vi "AudioTest.Config, Read_Write Microphone Test Setup.vi"(7 "Read(F)/Write(T)":bool, 8 "error in (no error)":errorcluster, 10 "Params":T6={"Devices"={"AudioOutName"="Line", "AudioInName"="HMD"}, "SweepParams"={"Duration"=2.0, "Amplitude"=1.0, "FreqStart"=20.0, "FreqEnd"=20000.0, "SampleRate"=44100.0, "StepCnt"=120, "FreqSpacing"=enum."Logarithmic", "Settling"={"Time"=0.0, "Cycles"=1.0}, "Measurement"={"Time"=0.001, "Cycles"=10.0}, "SyncPulseEn"=FALSE}, "DataFolder"=path "C:/MTE/Utah Core Audio Test/Data", "AvgLevelParams"={"Freq Start"=20.0, "Freq End"=20000.0}, "Limits"={"CoveredMicAttn_dB"=500.0, "AvgLevelLL_dBFS"=12000.0, "AvgLevelUL_dBFS"=44100.0, "FreqRespLim"=path "C:/MTE/Utah Core Audio Test/Config/Microphone Test Freq Response Limits.ini", "THDLim"=path "C:/MTE/Utah Core Audio Test/Config/Microphone Test THD Limits.ini"}, "SpeakerCalFile"=path "C:/MTE/Utah Core Audio Test/Config/Microphone Test Speaker Calibration.ini", "Volume"=0.0} {"SweepParams"."Measurement"."Cycles" min=5.0 max=1000.0 step=1.0; "SweepParams"."Measurement"."Time" min=0.0 max=5.0 step=0.0001 format="%.3f s"; "SweepParams"."Settling"."Cycles" min=0.0 max=100.0 step=0.5; "SweepParams"."Settling"."Time" min=0.0 max=5.0 step=0.0001 format="%.3f s"; "SweepParams"."StepCnt" min=1; "SweepParams"."Amplitude" min=0.0 max=1.0 step=0.1}, 11 "Config Folder":path=path "C:/MTE/Utah Core Audio Test/Config") -> (0 "error out":errorcluster, 2 "Params":T5={"Devices"={"AudioOutName"="Line", "AudioInName"="HMD"}, "SweepParams"={"Duration"=2.0, "Amplitude"=1.0, "FreqStart"=20.0, "FreqEnd"=20000.0, "SampleRate"=44100.0, "StepCnt"=120, "FreqSpacing"=enum."Logarithmic", "Settling"={"Time"=0.0, "Cycles"=1.0}, "Measurement"={"Time"=0.001, "Cycles"=10.0}, "SyncPulseEn"=FALSE}, "DataFolder"=path "C:/MTE/Utah Core Audio Test/Data", "AvgLevelParams"={"Freq Start"=20.0, "Freq End"=20000.0}, "BlockedMicLim"={"CoveredMicAttn_dB"=500.0, "AvgLevelLL_dBFS"=12000.0, "AvgLevelUL_dBFS"=44100.0, "FreqRespLim"=path "C:/MTE/Utah Core Audio Test/Config/Microphone Test Freq Response Limits.ini", "THDLim"=path "C:/MTE/Utah Core Audio Test/Config/Microphone Test THD Limits.ini"}, "SpeakerCalFile"=path "C:/MTE/Utah Core Audio Test/Config/Microphone Test Speaker Calibration.ini", "Volume"=0.0} {"SweepParams"."Measurement"."Cycles" min=5.0 max=1000.0 step=1.0; "SweepParams"."Measurement"."Time" min=0.0 max=5.0 step=0.0001 format="%.3f s"; "SweepParams"."Settling"."Cycles" min=0.0 max=100.0 step=0.5; "SweepParams"."Settling"."Time" min=0.0 max=5.0 step=0.0001 format="%.3f s"; "SweepParams"."StepCnt" min=1; "SweepParams"."Amplitude" min=0.0 max=1.0 step=0.1})   [LabVIEW 2018]
uses:
  TypeDefs/AudioTest.Config, Device ID.ctl
  TypeDefs/AudioTest.Config, Sine Sweep Params_V2.ctl
  TypeDefs/AudioTest.Config, Average Level Config.ctl
  TypeDefs/AudioTest.Config, Limits, Blocked Mic Check.ctl
  <vilib>/Utility/config.llb/Config Data RefNum.ctl
  Common/Utils/Config/INI/Config.INI, Read_Write, String.vi
  Common/Utils/Config/INI/Config.INI, Read_Write, Float.vi
  Common/Utils/Config/INI/Config.INI, Read_Write, Path.vi
  Common/Utils/Config/INI/Config.INI, Read_Write, Integer.vi
  Common/Utils/Config/INI/Config.INI, Read_Write, Boolean.vi
  <vilib>/Utility/config.llb/NI_LVConfig.lvlib
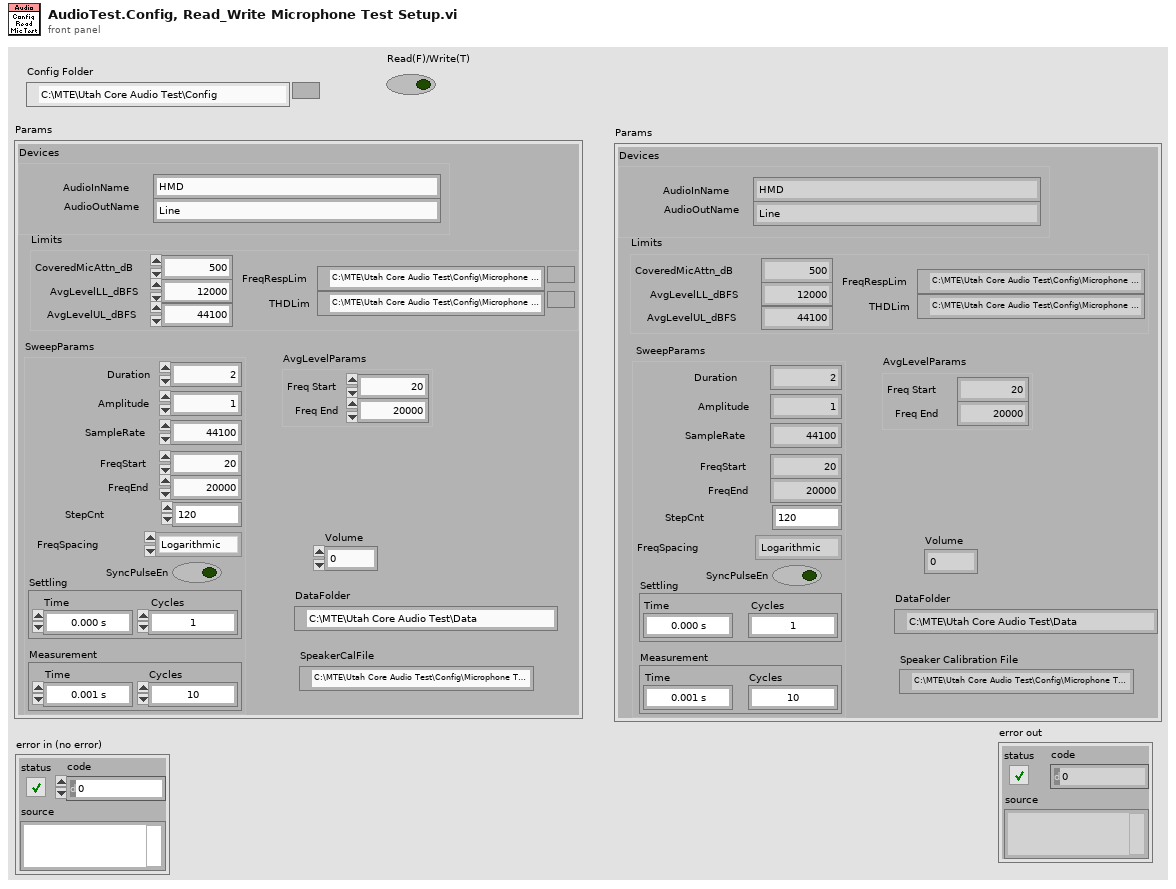
[diagram p1: front panel]
types:
  T1 = typedef "AudioTest.Config, Device ID.ctl" = cluster{"AudioOutName":string, "AudioInName":string}
  T2 = typedef "AudioTest.Config, Sine Sweep Params_V2.ctl" = cluster{"Duration":dbl, "Amplitude":dbl, "FreqStart":dbl, "FreqEnd":dbl, "SampleRate":dbl, "StepCnt":i32, "FreqSpacing":enum16{"Linear", "Logarithmic"}, "Settling":cluster{"Time":dbl, "Cycles":dbl}, "Measurement":cluster{"Time":dbl, "Cycles":dbl}, "SyncPulseEn":bool}
  T3 = typedef "AudioTest.Config, Average Level Config.ctl" = cluster{"Freq Start":dbl, "Freq End":dbl}
  T4 = typedef "AudioTest.Config, Limits, Blocked Mic Check.ctl" = cluster{"CoveredMicAttn_dB":dbl, "AvgLevelLL_dBFS":dbl, "AvgLevelUL_dBFS":dbl, "FreqRespLim":path, "THDLim":path}
  T5 = cluster{"Devices":T1, "SweepParams":T2, "DataFolder":path, "AvgLevelParams":T3, "BlockedMicLim":T4, "SpeakerCalFile":path, "Volume":dbl}
  T6 = cluster{"Devices":T1, "SweepParams":T2, "DataFolder":path, "AvgLevelParams":T3, "Limits":T4, "SpeakerCalFile":path, "Volume":dbl}
  T7 = typedef "NI_LVConfig.lvlib/Config Data RefNum.ctl" = refnum<k1>
  T8 = cluster{"FileRef":T7, "Params":cluster{"Devices":T1, "SweepParams":T2, "DataFolder":path, "AvgLevelParams":T3, "Limits":T4, "SpeakerCalFile":path, "Volume":dbl}, "Write":bool}
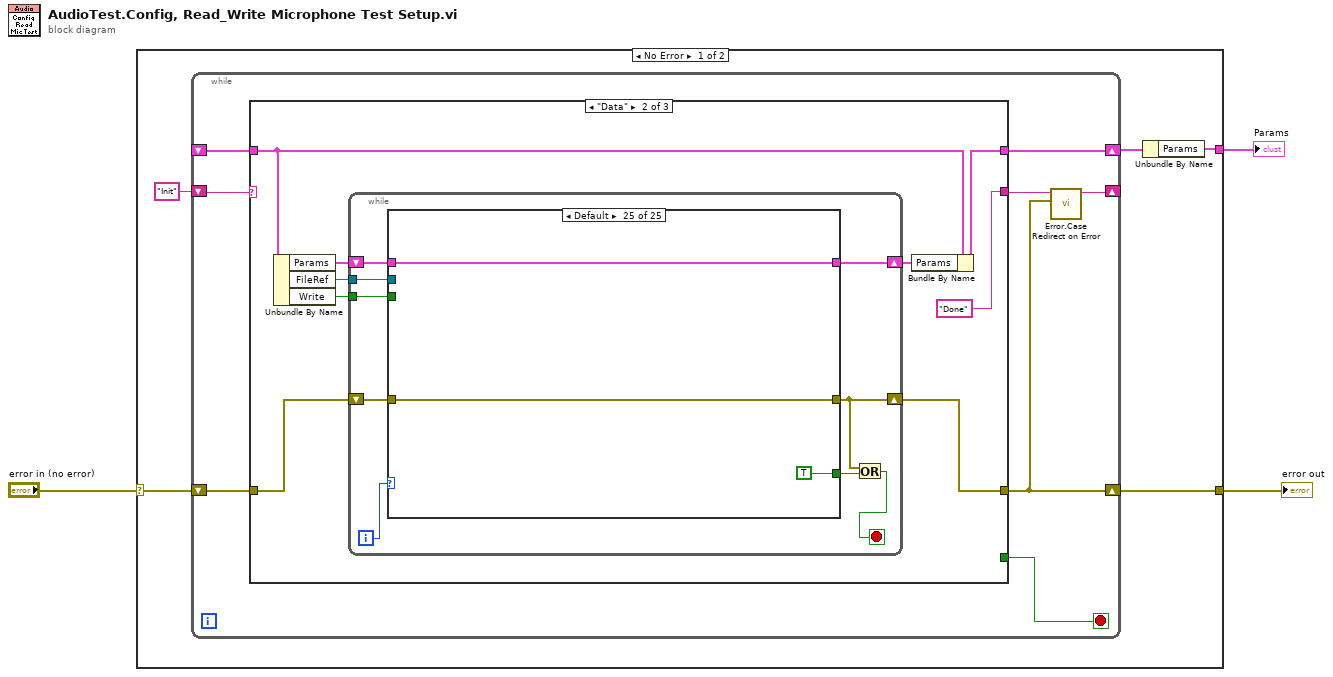
[diagram p0: block diagram]
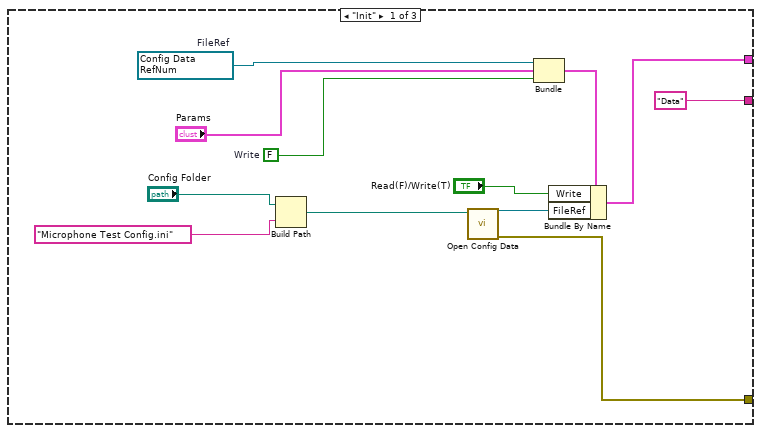
[diagram p2: hidden frame]
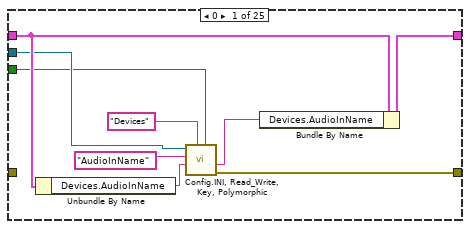
[diagram p3: hidden frame]
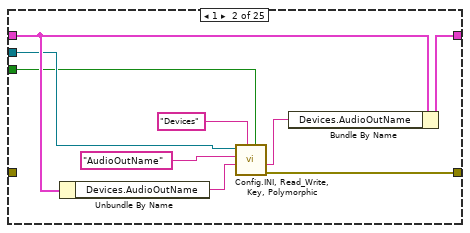
[diagram p4: hidden frame]
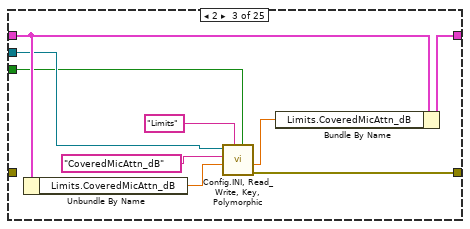
[diagram p5: hidden frame]
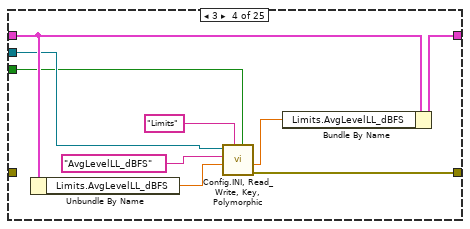
[diagram p6: hidden frame]
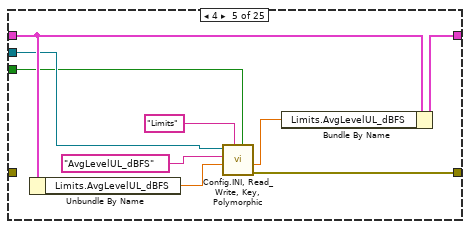
[diagram p7: hidden frame]
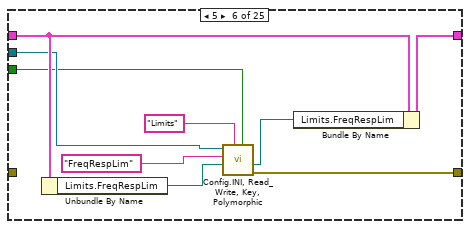
[diagram p8: hidden frame]
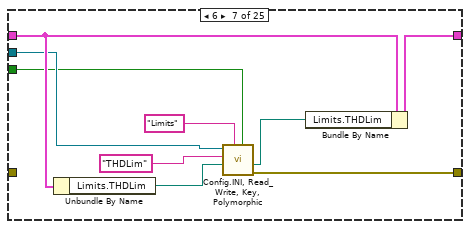
[diagram p9: hidden frame]
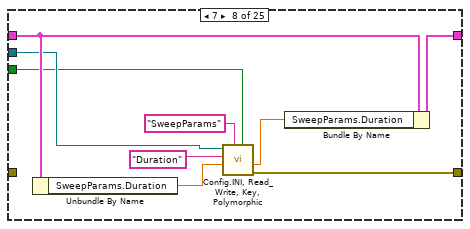
[diagram p10: hidden frame]
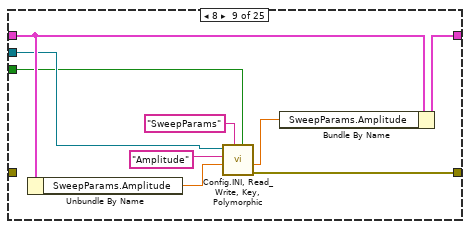
[diagram p11: hidden frame]
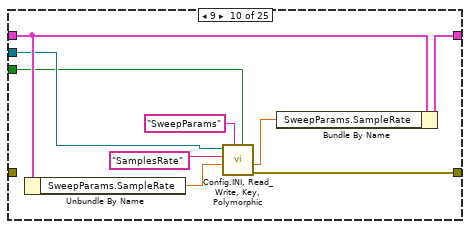
[diagram p12: hidden frame]
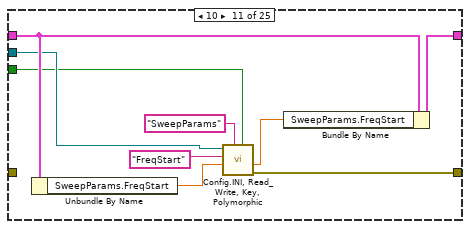
[diagram p13: hidden frame]
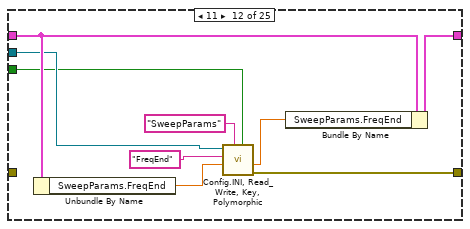
[diagram p14: hidden frame]
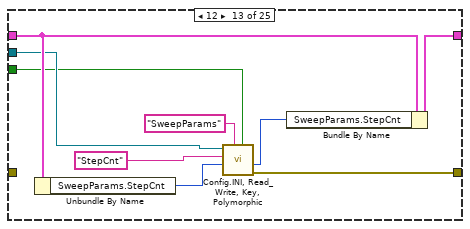
[diagram p15: hidden frame]
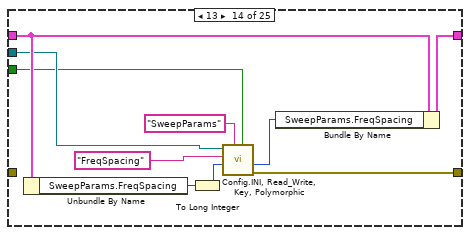
[diagram p16: hidden frame]
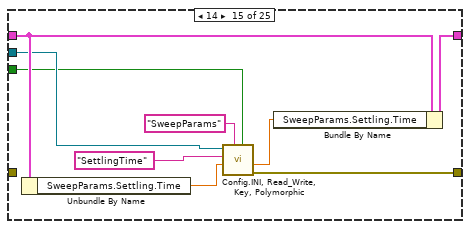
[diagram p17: hidden frame]
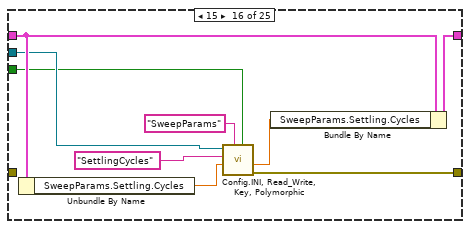
[diagram p18: hidden frame]
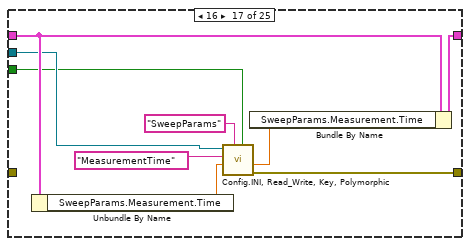
[diagram p19: hidden frame]
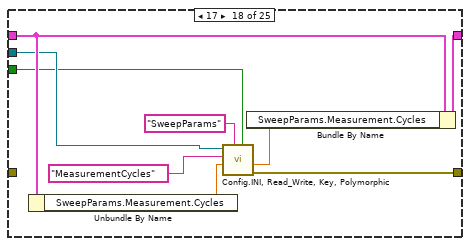
[diagram p20: hidden frame]
diagram:
  n1 = case shown="No Error" "error in (no error)" {
    selector: "error in (no error)" -> [w7 w273]
    tunnel: [w6 w273] -> w2
    tunnel: [w4 _] -> w1
    frame No Error {
      n2 = while {
        shift-right: [w10] -> _
        shift-left: "Init" -> [w16]
        shift-right: [w15] -> w5
        shift-left: _ -> [w9]
        shift-right: [w11] -> w6
        shift-left: w7 -> [w13]
        stop <- w14 stop-if-true
        n3 = case shown="\"Data\"" w16 {
          tunnel: ["Data" "Done" "Done"] -> w12
          tunnel: [w22 w34 w269] -> w15
          tunnel: [_ _ TRUE] -> w14
          tunnel: w13 -> [_ w30 w271]
          tunnel: [w20 w31 w271] -> w11
          tunnel: w9 -> [_ w33 w269]
          frame "Init" {
            w19 = FALSE  # Write
            w25 = T7 refnum items=["config data"]  # FileRef
            n4 = Build Path(base path="Config Folder", name or relative path="Microphone Test Config.ini") -> (appended path=w26:path)
            n5 = call <vilib>:"Open Config Data.vi"("configuration file path"=w26) -> ("error out"=w20:errorcluster, "refnum"=w21:T7)  [unwired: 8 in, 1 out]
            n6 = Bundle("FileRef"=w25, "Params"="Params", "Write"=w19) -> (w23:T8)  [unwired: 1 in]
            n7 = Bundle By Name(cluster=w23, "Write"="Read(F)/Write(T)", "FileRef"=w21) -> (w22:T8)
          }
          frame "Data" {
            n8 = Unbundle By Name(w33) -> ("Params"=w37:T6, "FileRef"=w36:T7, "Write"=w29:bool)
            n9 = while {
              shift-right: [w45] -> w35
              shift-left: w37 -> [w46]
              tunnel: w36 -> [w43]
              shift-right: [w42] -> w31
              shift-left: w30 -> [w41]
              tunnel: w29 -> [w38]
              i -> [w44]
              stop <- w39 stop-if-true
              n10 = case shown="Default" w44 {
                tunnel: w46 -> [w55 w64 w73 w82 w91 w100 w109 w118 w127 w136 w145 w154 w163 w173 w182 w191 w200 w209 w218 w227 w236 w245 w254 w263 w266]
                tunnel: [w54 w63 w72 w81 w90 w99 w108 w117 w126 w135 w144 w153 w162 w172 w181 w190 w199 w208 w217 w226 w235 w244 w253 w262 w266] -> w45
                tunnel: w43 -> [w50 w59 w68 w77 w86 w95 w104 w113 w122 w131 w140 w149 w158 w169 w178 w187 w196 w205 w213 w223 w231 w240 w249 w258 _]
                tunnel: [w49 w58 w67 w76 w85 w94 w103 w112 w121 w130 w139 w148 w157 w168 w177 w186 w195 w204 w212 w222 w230 w239 w248 w257 w265] -> w42
                tunnel: w41 -> [_ _ _ _ _ _ _ _ _ _ _ _ _ _ _ _ _ _ _ _ _ _ _ _ w265]
                tunnel: [_ _ _ _ _ _ _ _ _ _ _ _ _ _ _ _ _ _ _ _ _ _ _ _ TRUE] -> w40
                tunnel: w38 -> [w47 w56 w65 w74 w83 w92 w101 w110 w119 w128 w137 w146 w155 w167 w176 w185 w194 w203 w210 w221 w228 w237 w246 w255 _]
                frame 0 {
                  n11 = Unbundle By Name(w55) -> ("Devices.AudioInName"=w51:string)
                  n12 = call-poly "Config.INI, Read_Write, Key, Polymorphic.vi"("Read(F)/Write(T)"=w47, "Section"="Devices", "Value/DefaultValue"=w51, "Key"="AudioInName", "refnum"=w50) -> ("error out"=w49:errorcluster, "Value Out"=w48:string)  [unwired: 3 in, 2 out]
                  n13 = Bundle By Name(cluster=w55, "Devices.AudioInName"=w48) -> (w54:T6)
                }
                frame 1 {
                  n14 = Unbundle By Name(w64) -> ("Devices.AudioOutName"=w60:string)
                  n15 = call-poly "Config.INI, Read_Write, Key, Polymorphic.vi"("Read(F)/Write(T)"=w56, "Section"="Devices", "Value/DefaultValue"=w60, "Key"="AudioOutName", "refnum"=w59) -> ("error out"=w58:errorcluster, "Value Out"=w57:string)  [unwired: 3 in, 2 out]
                  n16 = Bundle By Name(cluster=w64, "Devices.AudioOutName"=w57) -> (w63:T6)
                }
                frame 2 {
                  n17 = Unbundle By Name(w73) -> ("Limits.CoveredMicAttn_dB"=w69:dbl)
                  n18 = call-poly "Config.INI, Read_Write, Key, Polymorphic.vi"("Read(F)/Write(T)"=w65, "Section"="Limits", "Value/DefaultValue"=w69, "Key"="CoveredMicAttn_dB", "refnum"=w68) -> ("error out"=w67:errorcluster, "Value Out"=w66:dbl)  [unwired: 3 in, 2 out]
                  n19 = Bundle By Name(cluster=w73, "Limits.CoveredMicAttn_dB"=w66) -> (w72:T6)
                }
                frame 3 {
                  n20 = Unbundle By Name(w82) -> ("Limits.AvgLevelLL_dBFS"=w78:dbl)
                  n21 = call-poly "Config.INI, Read_Write, Key, Polymorphic.vi"("Read(F)/Write(T)"=w74, "Section"="Limits", "Value/DefaultValue"=w78, "Key"="AvgLevelLL_dBFS", "refnum"=w77) -> ("error out"=w76:errorcluster, "Value Out"=w75:dbl)  [unwired: 3 in, 2 out]
                  n22 = Bundle By Name(cluster=w82, "Limits.AvgLevelLL_dBFS"=w75) -> (w81:T6)
                }
                frame 4 {
                  n23 = Unbundle By Name(w91) -> ("Limits.AvgLevelUL_dBFS"=w87:dbl)
                  n24 = call-poly "Config.INI, Read_Write, Key, Polymorphic.vi"("Read(F)/Write(T)"=w83, "Section"="Limits", "Value/DefaultValue"=w87, "Key"="AvgLevelUL_dBFS", "refnum"=w86) -> ("error out"=w85:errorcluster, "Value Out"=w84:dbl)  [unwired: 3 in, 2 out]
                  n25 = Bundle By Name(cluster=w91, "Limits.AvgLevelUL_dBFS"=w84) -> (w90:T6)
                }
                frame 5 {
                  n26 = Unbundle By Name(w100) -> ("Limits.FreqRespLim"=w96:path)
                  n27 = call-poly "Config.INI, Read_Write, Key, Polymorphic.vi"("Read(F)/Write(T)"=w92, "Section"="Limits", "Value/DefaultValue"=w96, "Key"="FreqRespLim", "refnum"=w95) -> ("error out"=w94:errorcluster, "Value Out"=w93:path)  [unwired: 3 in, 2 out]
                  n28 = Bundle By Name(cluster=w100, "Limits.FreqRespLim"=w93) -> (w99:T6)
                }
                frame 6 {
                  n29 = Unbundle By Name(w109) -> ("Limits.THDLim"=w105:path)
                  n30 = call-poly "Config.INI, Read_Write, Key, Polymorphic.vi"("Read(F)/Write(T)"=w101, "Section"="Limits", "Value/DefaultValue"=w105, "Key"="THDLim", "refnum"=w104) -> ("error out"=w103:errorcluster, "Value Out"=w102:path)  [unwired: 3 in, 2 out]
                  n31 = Bundle By Name(cluster=w109, "Limits.THDLim"=w102) -> (w108:T6)
                }
                frame 7 {
                  n32 = Unbundle By Name(w118) -> ("SweepParams.Duration"=w114:dbl)
                  n33 = call-poly "Config.INI, Read_Write, Key, Polymorphic.vi"("Read(F)/Write(T)"=w110, "Section"="SweepParams", "Value/DefaultValue"=w114, "Key"="Duration", "refnum"=w113) -> ("error out"=w112:errorcluster, "Value Out"=w111:dbl)  [unwired: 3 in, 2 out]
                  n34 = Bundle By Name(cluster=w118, "SweepParams.Duration"=w111) -> (w117:T6)
                }
                frame 8 {
                  n35 = Unbundle By Name(w127) -> ("SweepParams.Amplitude"=w123:dbl)
                  n36 = call-poly "Config.INI, Read_Write, Key, Polymorphic.vi"("Read(F)/Write(T)"=w119, "Section"="SweepParams", "Value/DefaultValue"=w123, "Key"="Amplitude", "refnum"=w122) -> ("error out"=w121:errorcluster, "Value Out"=w120:dbl)  [unwired: 3 in, 2 out]
                  n37 = Bundle By Name(cluster=w127, "SweepParams.Amplitude"=w120) -> (w126:T6)
                }
                frame 9 {
                  n38 = Unbundle By Name(w136) -> ("SweepParams.SampleRate"=w132:dbl)
                  n39 = call-poly "Config.INI, Read_Write, Key, Polymorphic.vi"("Read(F)/Write(T)"=w128, "Section"="SweepParams", "Value/DefaultValue"=w132, "Key"="SamplesRate", "refnum"=w131) -> ("error out"=w130:errorcluster, "Value Out"=w129:dbl)  [unwired: 3 in, 2 out]
                  n40 = Bundle By Name(cluster=w136, "SweepParams.SampleRate"=w129) -> (w135:T6)
                }
                frame 10 {
                  n41 = Unbundle By Name(w145) -> ("SweepParams.FreqStart"=w141:dbl)
                  n42 = call-poly "Config.INI, Read_Write, Key, Polymorphic.vi"("Read(F)/Write(T)"=w137, "Section"="SweepParams", "Value/DefaultValue"=w141, "Key"="FreqStart", "refnum"=w140) -> ("error out"=w139:errorcluster, "Value Out"=w138:dbl)  [unwired: 3 in, 2 out]
                  n43 = Bundle By Name(cluster=w145, "SweepParams.FreqStart"=w138) -> (w144:T6)
                }
                frame 11 {
                  n44 = Unbundle By Name(w154) -> ("SweepParams.FreqEnd"=w150:dbl)
                  n45 = call-poly "Config.INI, Read_Write, Key, Polymorphic.vi"("Read(F)/Write(T)"=w146, "Section"="SweepParams", "Value/DefaultValue"=w150, "Key"="FreqEnd", "refnum"=w149) -> ("error out"=w148:errorcluster, "Value Out"=w147:dbl)  [unwired: 3 in, 2 out]
                  n46 = Bundle By Name(cluster=w154, "SweepParams.FreqEnd"=w147) -> (w153:T6)
                }
                frame 12 {
                  n47 = Unbundle By Name(w163) -> ("SweepParams.StepCnt"=w159:i32)
                  n48 = call-poly "Config.INI, Read_Write, Key, Polymorphic.vi"("Read(F)/Write(T)"=w155, "Section"="SweepParams", "Value/DefaultValue"=w159, "Key"="StepCnt", "refnum"=w158) -> ("error out"=w157:errorcluster, "Value Out"=w156:i32)  [unwired: 3 in, 2 out]
                  n49 = Bundle By Name(cluster=w163, "SweepParams.StepCnt"=w156) -> (w162:T6)
                }
                frame 13 {
                  n50 = Unbundle By Name(w173) -> ("SweepParams.FreqSpacing"=w165:enum16{"Linear", "Logarithmic"})
                  n51 = To Long Integer(number=w165) -> (32bit integer=w166:i32)
                  n52 = call-poly "Config.INI, Read_Write, Key, Polymorphic.vi"("Read(F)/Write(T)"=w167, "Section"="SweepParams", "Value/DefaultValue"=w166, "Key"="FreqSpacing", "refnum"=w169) -> ("error out"=w168:errorcluster, "Value Out"=w164:i32)  [unwired: 3 in, 2 out]
                  n53 = Bundle By Name(cluster=w173, "SweepParams.FreqSpacing"=w164) -> (w172:T6)
                }
                frame 14 {
                  n54 = Unbundle By Name(w182) -> ("SweepParams.Settling.Time"=w174:dbl)
                  n55 = call-poly "Config.INI, Read_Write, Key, Polymorphic.vi"("Read(F)/Write(T)"=w176, "Section"="SweepParams", "Value/DefaultValue"=w174, "Key"="SettlingTime", "refnum"=w178) -> ("error out"=w177:errorcluster, "Value Out"=w175:dbl)  [unwired: 3 in, 2 out]
                  n56 = Bundle By Name(cluster=w182, "SweepParams.Settling.Time"=w175) -> (w181:T6)
                }
                frame 15 {
                  n57 = Unbundle By Name(w191) -> ("SweepParams.Settling.Cycles"=w183:dbl)
                  n58 = call-poly "Config.INI, Read_Write, Key, Polymorphic.vi"("Read(F)/Write(T)"=w185, "Section"="SweepParams", "Value/DefaultValue"=w183, "Key"="SettlingCycles", "refnum"=w187) -> ("error out"=w186:errorcluster, "Value Out"=w184:dbl)  [unwired: 3 in, 2 out]
                  n59 = Bundle By Name(cluster=w191, "SweepParams.Settling.Cycles"=w184) -> (w190:T6)
                }
                frame 16 {
                  n60 = Unbundle By Name(w200) -> ("SweepParams.Measurement.Time"=w192:dbl)
                  n61 = call-poly "Config.INI, Read_Write, Key, Polymorphic.vi"("Read(F)/Write(T)"=w194, "Section"="SweepParams", "Value/DefaultValue"=w192, "Key"="MeasurementTime", "refnum"=w196) -> ("error out"=w195:errorcluster, "Value Out"=w193:dbl)  [unwired: 3 in, 2 out]
                  n62 = Bundle By Name(cluster=w200, "SweepParams.Measurement.Time"=w193) -> (w199:T6)
                }
                frame 17 {
                  n63 = Unbundle By Name(w209) -> ("SweepParams.Measurement.Cycles"=w201:dbl)
                  n64 = call-poly "Config.INI, Read_Write, Key, Polymorphic.vi"("Read(F)/Write(T)"=w203, "Section"="SweepParams", "Value/DefaultValue"=w201, "Key"="MeasurementCycles", "refnum"=w205) -> ("error out"=w204:errorcluster, "Value Out"=w202:dbl)  [unwired: 3 in, 2 out]
                  n65 = Bundle By Name(cluster=w209, "SweepParams.Measurement.Cycles"=w202) -> (w208:T6)
                }
                frame 18 {
                  n66 = Unbundle By Name(w218) -> ("Volume"=w214:dbl)
                  n67 = call-poly "Config.INI, Read_Write, Key, Polymorphic.vi"("Read(F)/Write(T)"=w210, "Section"="SweepParams", "Value/DefaultValue"=w214, "Key"="Volume", "refnum"=w213) -> ("error out"=w212:errorcluster, "Value Out"=w211:dbl)  [unwired: 3 in, 2 out]
                  n68 = Bundle By Name(cluster=w218, "Volume"=w211) -> (w217:T6)
                }
                frame 19 {
                  n69 = Unbundle By Name(w227) -> ("SweepParams.SyncPulseEn"=w220:bool)
                  n70 = call-poly "Config.INI, Read_Write, Key, Polymorphic.vi"("Read(F)/Write(T)"=w221, "Section"="SweepParams", "Value/DefaultValue"=w220, "Key"="SyncPulseEn", "refnum"=w223) -> ("error out"=w222:errorcluster, "Value Out"=w219:bool)  [unwired: 3 in, 2 out]
                  n71 = Bundle By Name(cluster=w227, "SweepParams.SyncPulseEn"=w219) -> (w226:T6)
                }
                frame 20 {
                  n72 = Unbundle By Name(w236) -> ("DataFolder"=w232:path)
                  n73 = call-poly "Config.INI, Read_Write, Key, Polymorphic.vi"("Read(F)/Write(T)"=w228, "Section"="Paths", "Value/DefaultValue"=w232, "Key"="DefaultDataFolder", "refnum"=w231) -> ("error out"=w230:errorcluster, "Value Out"=w229:path)  [unwired: 3 in, 2 out]
                  n74 = Bundle By Name(cluster=w236, "DataFolder"=w229) -> (w235:T6)
                }
                frame 21 {
                  n75 = Unbundle By Name(w245) -> ("SpeakerCalFile"=w241:path)
                  n76 = call-poly "Config.INI, Read_Write, Key, Polymorphic.vi"("Read(F)/Write(T)"=w237, "Section"="Calibration", "Value/DefaultValue"=w241, "Key"="SpeakerCalFile", "refnum"=w240) -> ("error out"=w239:errorcluster, "Value Out"=w238:path)  [unwired: 3 in, 2 out]
                  n77 = Bundle By Name(cluster=w245, "SpeakerCalFile"=w238) -> (w244:T6)
                }
                frame 22 {
                  n78 = Unbundle By Name(w254) -> ("AvgLevelParams.Freq Start"=w250:dbl)
                  n79 = call-poly "Config.INI, Read_Write, Key, Polymorphic.vi"("Read(F)/Write(T)"=w246, "Section"="AvgLevelParams", "Value/DefaultValue"=w250, "Key"="FreqStart", "refnum"=w249) -> ("error out"=w248:errorcluster, "Value Out"=w247:dbl)  [unwired: 3 in, 2 out]
                  n80 = Bundle By Name(cluster=w254, "AvgLevelParams.Freq Start"=w247) -> (w253:T6)
                }
                frame 23 {
                  n81 = Unbundle By Name(w263) -> ("AvgLevelParams.Freq End"=w259:dbl)
                  n82 = call-poly "Config.INI, Read_Write, Key, Polymorphic.vi"("Read(F)/Write(T)"=w255, "Section"="AvgLevelParams", "Value/DefaultValue"=w259, "Key"="FreqEnd", "refnum"=w258) -> ("error out"=w257:errorcluster, "Value Out"=w256:dbl)  [unwired: 3 in, 2 out]
                  n83 = Bundle By Name(cluster=w263, "AvgLevelParams.Freq End"=w256) -> (w262:T6)
                }
                frame Default {
                }
              }
              n84 = Or(x=w42, y=w40) -> (x .or. y?=w39:bool)
            }
            n85 = Bundle By Name(cluster=w33, "Params"=w35) -> (w34:T8)
          }
          frame "Done", Default {
            n86 = Unbundle By Name(w269) -> ("FileRef"=w268:T7)
            n87 = call <vilib>:"Close Config Data.vi"("refnum"=w268) -> ("error out"=w267:errorcluster)  [unwired: 9 in, 1 out]
            n88 = call <vilib>:"Clear Errors.vi"("error in (no error)"=w267) -> ()  [unwired: 5 in, 2 out]
          }
        }
        n89 = call "Error.Case Redirect on Error.vi"("error in"=w11, "Next Case"=w12) -> ("Next Case Out"=w10:string)  [unwired: 9 in]
      }
      n90 = Unbundle By Name(w5) -> ("Params"=w4:T6)
    }
    frame Error {
    }
  }
  "error out" <- w2
  "Params" <- w1
